vi "Create Getter Case in Message Handler.vi"(8 "error in (no error)":errorcluster, 11 "Setter Generator In":refnum<class "API VI Generator.lvclass">) -> (0 "error out":errorcluster, 3 "Setter Generator Out":refnum<class "API VI Generator.lvclass">)   [LabVIEW 2020, in "Method Generation.lvlib" / "API VI Generator.lvclass"]
uses:
  API VI Generator.lvclass
  <vilib>/Utility/traverseref.llb/TRef TravTarget.ctl
  API VI Generator.lvclass/API VI Generator.ctl
  <vilib>/Utility/traverseref.llb/VI Scripting - Traverse.lvlib
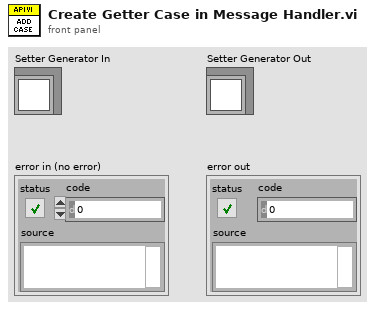
[diagram p1: front panel]
types:
  T1 = typedef "TRef TravTarget.ctl" = enum16{"FP", "BD", "Other"}
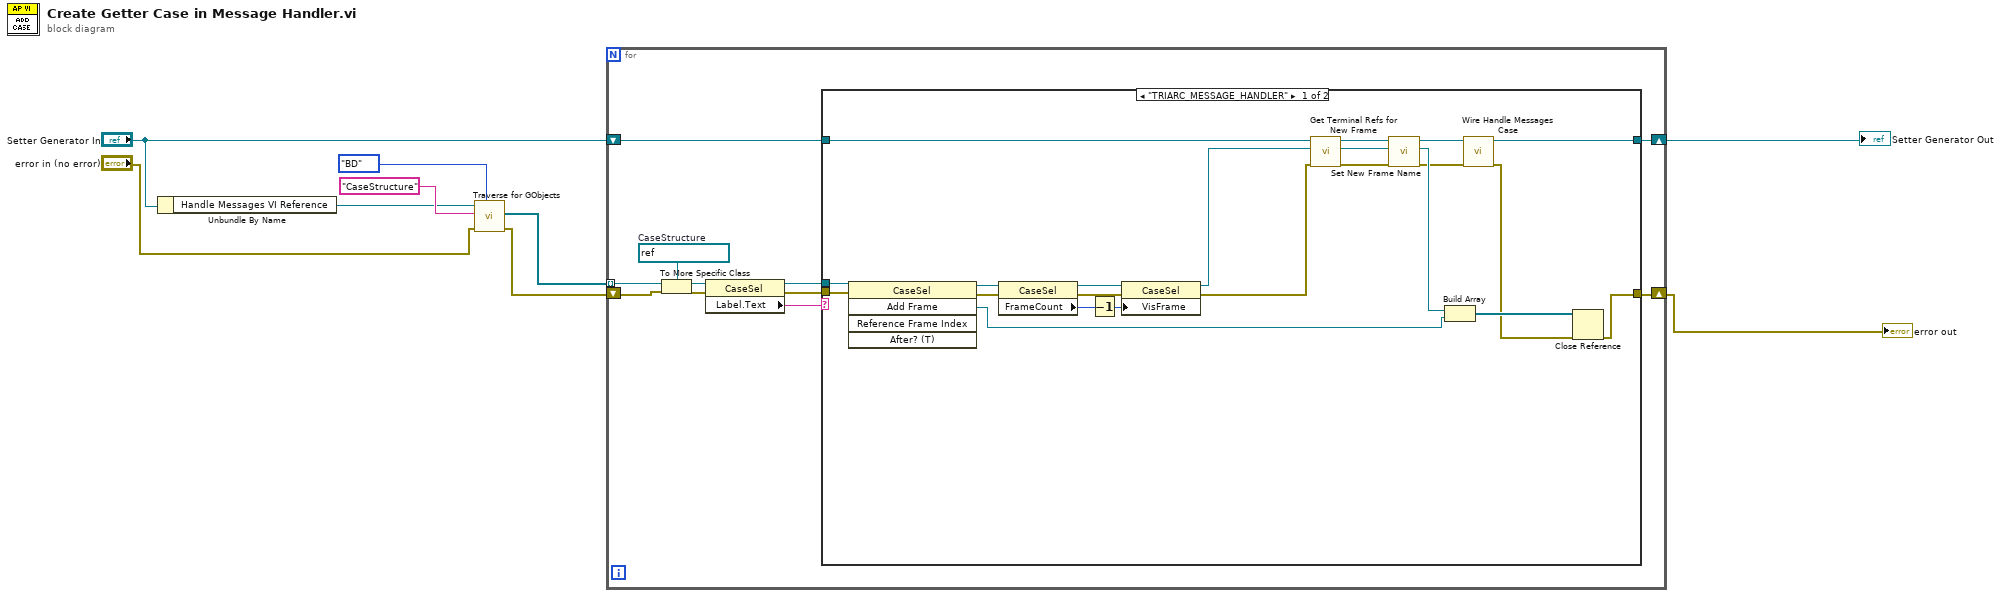
[diagram p0: block diagram]
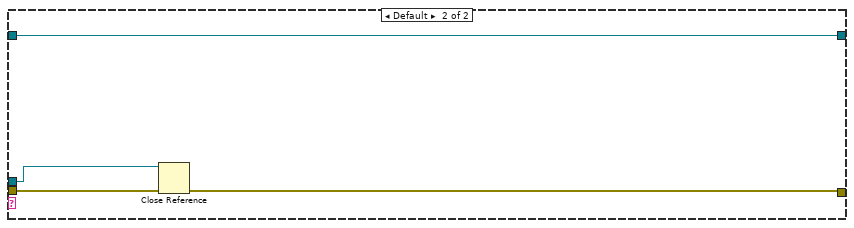
[diagram p2: hidden frame]
diagram:
  n1 = Unbundle By Name("Setter Generator In") -> ("Handle Messages VI Reference"=w1:refnum<vi>)
  n2 = call <vilib>:"Traverse for GObjects.vi"("Traverse Target"=TRef_TravTarget."BD", "error in (no error)"="error in (no error)", "Class Name"="CaseStructure", "VI Refnum"=w1) -> ("error out"=w2:errorcluster, "References"=w4:refnum<vi>[])  [unwired: 4 in, 2 out]
  n3 = for {
    tunnel: w4 -> [w18] mode=indexing
    shift-right: [w12] -> w3
    shift-left: w2 -> [w15]
    shift-right: [w10] -> w6
    shift-left: "Setter Generator In" -> [w11]
    w14 = refnum<vi> refnum  # CaseStructure
    n4 = To More Specific Class(target class=w14, reference=w18, error in=w15) -> (specific class reference=w17:refnum<vi>, error out=w16:errorcluster)
    n5 = property class="CaseSel"(reference=w17, error in=w16) -> (reference out=w19:refnum<vi>, error out=w13:errorcluster, "Label.Text"=w20:string)
    n6 = case shown="\"TRIARC_MESSAGE_HANDLER\"" w20 {
      tunnel: w19 -> [w42 w46]
      tunnel: w13 -> [w41 w45]
      tunnel: [w35 w44] -> w12
      tunnel: w11 -> [w40 w43]
      tunnel: [w34 w43] -> w10
      frame "TRIARC_MESSAGE_HANDLER" {
        n7 = invoke class="CaseSel" method="Add Frame"(reference=w42, error in=w41) -> (reference out=w26:refnum<vi>, error out=w23:errorcluster, "Add Frame"=w21:refnum<vi>)  [unwired: 3 in, 2 out]
        n8 = property class="CaseSel"(reference=w26, error in=w23) -> (reference out=w25:refnum<vi>, error out=w24:errorcluster, "FrameCount"=w27:i32)
        n9 = Decrement(x=w27) -> (x-1=w22:i32)
        n10 = property class="CaseSel"(reference=w25, error in=w24, "VisFrame"=w22) -> (reference out=w39:refnum<vi>, error out=w38:errorcluster)
        n11 = call "Get Terminal Refs for New Frame.vi"("error in (no error)"=w38, "Case Structure Ref"=w39, "Setter Generator In"=w40) -> ("error out"=w30:errorcluster, "reference out"=w32:refnum<vi>, "Setter Generator Out"=w37:refnum<class "API VI Generator.lvclass">)  [unwired: 6 in]
        n12 = call "Set New Frame Name.vi"("error in (no error)"=w30, "reference in"=w32, "Setter Generator In"=w37) -> ("error out"=w29:errorcluster, "reference out"=w31:refnum<vi>, "Setter Generator Out"=w28:refnum<class "API VI Generator.lvclass">)  [unwired: 6 in]
        n13 = Build Array(w31, w21) -> (w36:refnum<vi>[])
        n14 = call "Wire Handle Messages Case.vi"("error in (no error)"=w29, "Setter Generator In"=w28) -> ("error out"=w33:errorcluster, "Setter Generator Out"=w34:refnum<class "API VI Generator.lvclass">)  [unwired: 8 in]
        n15 = Close Reference(reference=w36, error in (no error)=w33) -> (error out=w35:errorcluster)
      }
      frame Default {
        n16 = Close Reference(reference=w46, error in (no error)=w45) -> (error out=w44:errorcluster)
      }
    }
  }
  "Setter Generator Out" <- w6
  "error out" <- w3
